vi "TEG P116x2w_Write_Auto.vi"(7 "MaxOutput":T1={"Ch1"=100.0, "Ch2"=100.0}, 8 "error in (no error)":errorcluster, 9 "RateSP":T1, 10 "NuevoSP":T1, 11 "Comunicaciones":T2={"Alicats"="ASRL6::INSTR", "Alic"=FALSE, "eValve"="ASRL6::INSTR", "eval"=FALSE, "Eurotherm"="ASRL6::INSTR", "euro"=FALSE, "Cell GAS"="ASRL6::INSTR", "cgas"=FALSE, "Cell H2S"="ASRL6::INSTR", "ch2s"=FALSE}) -> (0 "error out":errorcluster, 1 "RateSP(C/min) 2":T1, 2 "NuevoSP(C) 2":T1, 3 "MaxOutput 2":T1)   [LabVIEW 2017]
uses:
  2xP116.ctl
  REACTOR_COMUNICACIONES.ctl
  Eurotherm_2023_Module.ctl
  REACTOR_GLOBALES.vi
panel:
  out "Temp":T1
  in  "Cancel":bool
  in  "Write":bool
  out "Enable(T)":bool=TRUE
  out "VISA Promux":refnum<visa-resource-name>
  in  "Delay Time (s)":dbl=0.1
  # "Programando controladores P116"
  # "C"
  # "%"
  # "CALOR"
  # "C/min"
  # "C"
  # "%"
  # "FRIO"
  # "C/min"
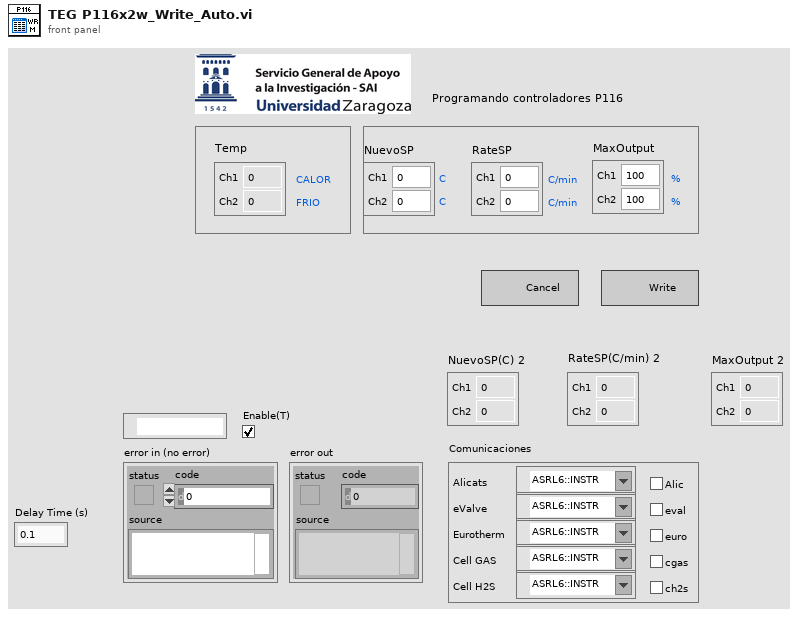
[diagram p1: front panel]
types:
  T1 = typedef "2xP116.ctl" = cluster{"Ch1":dbl, "Ch2":dbl}
  T2 = typedef "REACTOR_COMUNICACIONES.ctl" = cluster{"Alicats":refnum<visa-resource-name>, "Alic":bool, "eValve":refnum<visa-resource-name>, "eval":bool, "Eurotherm":refnum<visa-resource-name>, "euro":bool, "Cell GAS":refnum<visa-resource-name>, "cgas":bool, "Cell H2S":refnum<visa-resource-name>, "ch2s":bool}
  T3 = typedef "TEG P116x2w.ctl" = cluster{"TargetSP":T1, "WorkingSP":T1, "Temperatura":T1, "Error":bool, "Date":string, "Delay(s)":dbl, "RateSP":T1, "Potencia":T1, "Potencia max":T1}
  T4 = typedef "Eurotherm_2023_Module.ctl" = enum16{"Initialize", "Write setpoint", "Read data", "Write ramp rate", "Set constante proporcional", "Set constante integral", "Set constante diferencial", "Set ouput limit LOW", "Set ouput limit HIGH", "Shutdown"}
  T5 = enum16{"Add 1", "Add 2", "Add 3", "Add 10", "Add 11", "Add 12", "Add 13"}[]
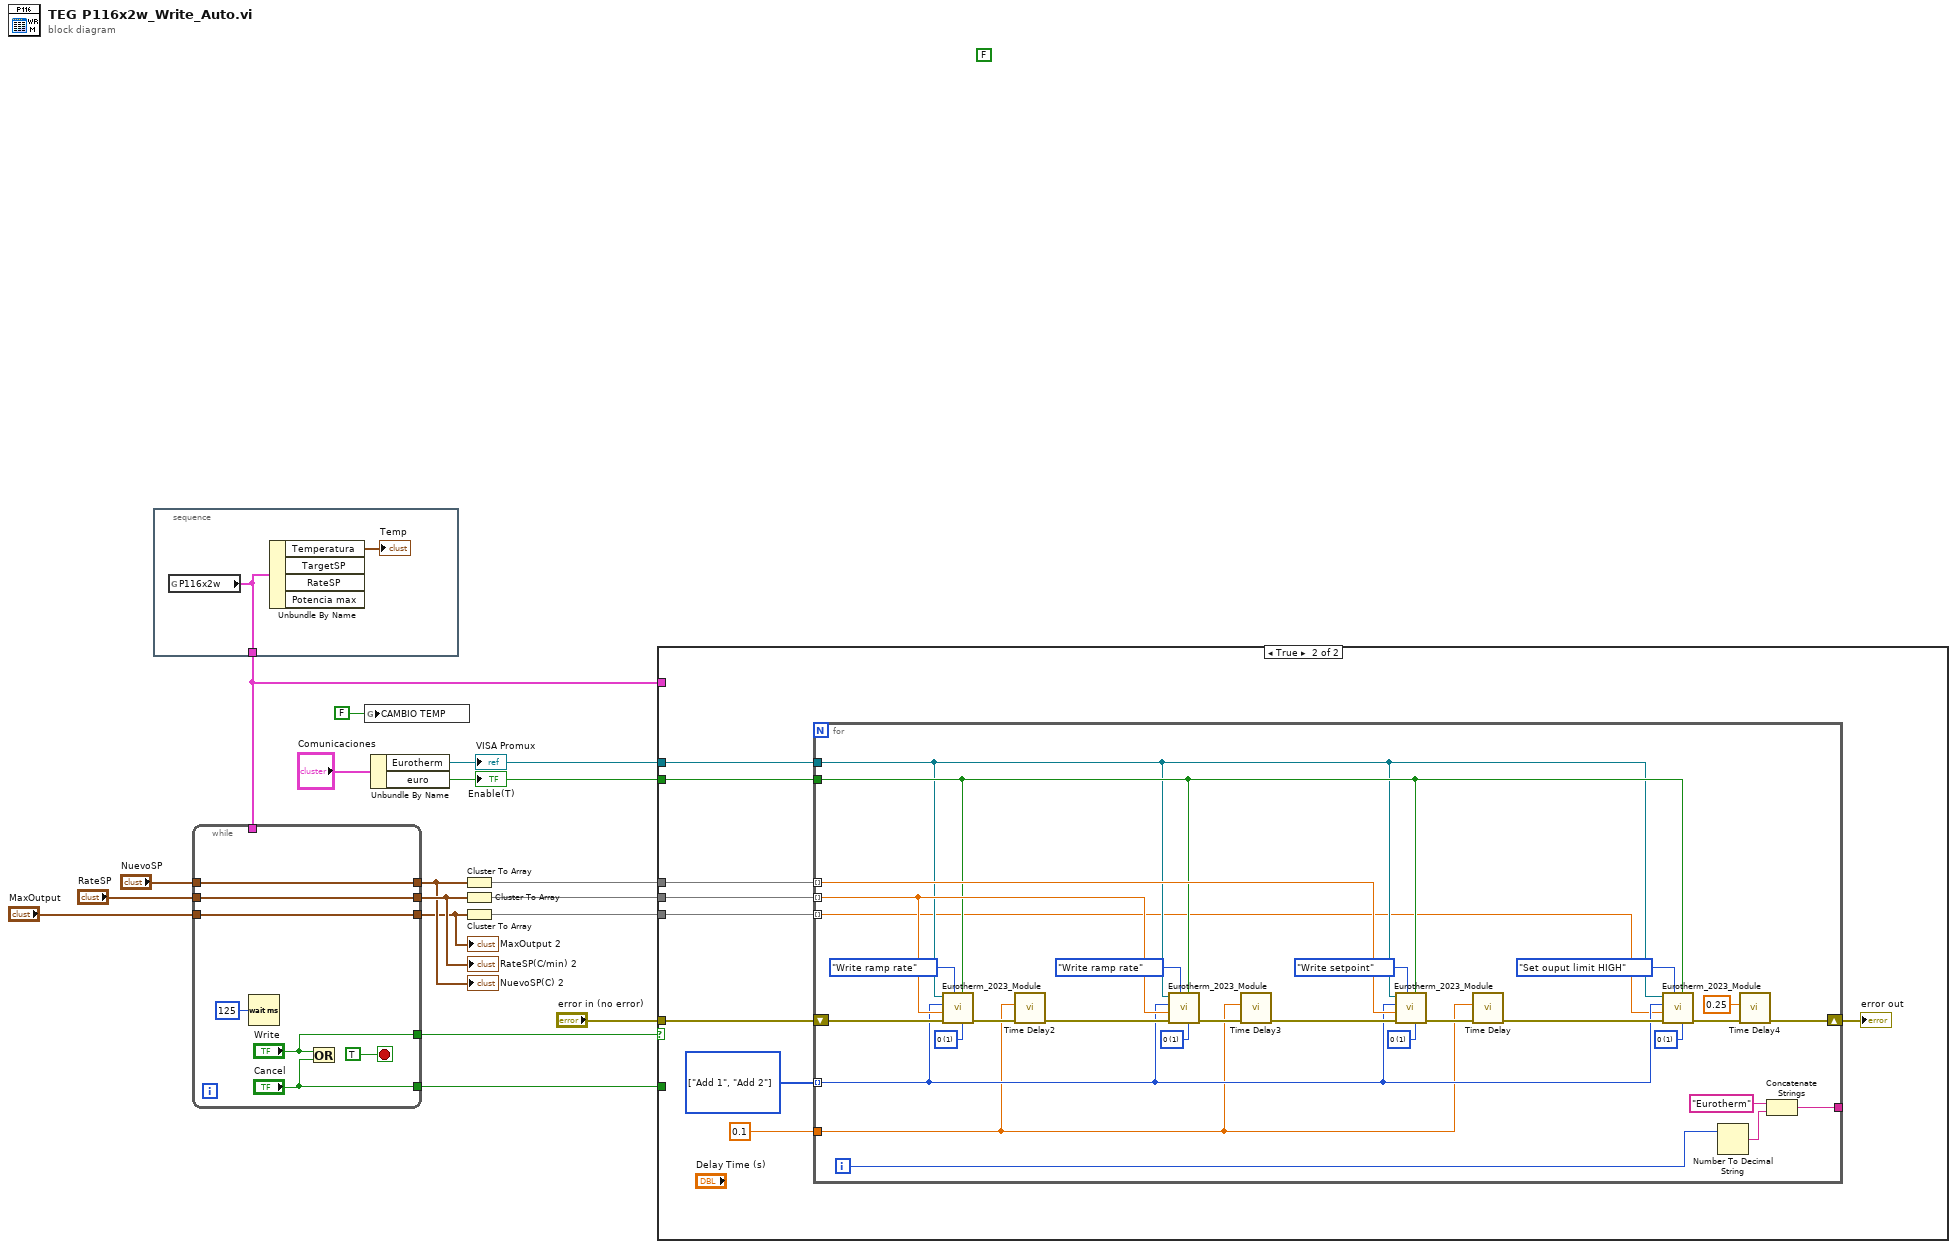
[diagram p0: block diagram]
diagram:
  (unwired) FALSE
  n1 = stacked-sequence {
    tunnel: [w18] -> w9
    frame #0 {
      n2 = global read "REACTOR_GLOBALES.vi" "P116x2w"() -> (w18:T3)
      n3 = Unbundle By Name(w18) -> ("Temperatura"=→"Temp":T1)  [unwired: 3 out]
    }
  }
  n4 = while {
    tunnel: ["Cancel"] -> w16
    tunnel: [w23] -> w5
    tunnel: [w22] -> w8
    tunnel: ["Write"] -> w12
    tunnel: w9 -> [_]
    tunnel: [w21] -> w4
    tunnel: "NuevoSP" -> [w23]
    tunnel: "RateSP" -> [w22]
    tunnel: "MaxOutput" -> [w21]
    stop <- TRUE stop-if-true
    n5 = Wait (ms)(milliseconds to wait=u32 125) -> ()  [unwired: 1 out]
    n6 = Or(x="Write", y="Cancel") -> ()  [unwired: 1 out]
  }
  "NuevoSP(C) 2" <- w5
  "RateSP(C/min) 2" <- w8
  "MaxOutput 2" <- w4
  n7 = global write "REACTOR_GLOBALES.vi" "CAMBIO TEMP"(FALSE ("ChangeT")) -> ()
  n8 = Unbundle By Name("Comunicaciones") -> ("Eurotherm"=w10:refnum<visa-resource-name>, "euro"=w17:bool)
  "Enable(T)" <- w17
  "VISA Promux" <- w10
  n9 = Cluster To Array(cluster=w5) -> (array=w14:dbl[])
  n10 = Cluster To Array(cluster=w8) -> (array=w13:dbl[])
  n11 = Cluster To Array(cluster=w4) -> (array=w6:dbl[])
  n12 = case shown="True" w12 {
    tunnel: w17 -> [_ w34]
    tunnel: w16 -> [_ _]
    tunnel: "error in (no error)" -> [_ w32]
    tunnel: w14 -> [_ w30]
    tunnel: w13 -> [_ w31]
    tunnel: w10 -> [_ w35]
    tunnel: w9 -> [_ _]
    tunnel: w6 -> [_ w28]
    frame False {
    }
    frame True {
      w29 = T5 [enum."Add 1", enum."Add 2"] items=["Add 1", "Add 2", "Add 3", "Add 10", "Add 11", "Add 12", "Add 13"]
      n13 = for {
        shift-right: [w42] -> w33
        shift-left: w32 -> [w59]
        tunnel: [w62] -> _
        tunnel: w30 -> [w58] mode=indexing
        tunnel: w31 -> [w47] mode=indexing
        tunnel: w35 -> [w40]
        tunnel: w34 -> [w41]
        tunnel: w29 -> [w39] mode=indexing
        tunnel: w28 -> [w36] mode=indexing
        tunnel: 0.1 ("Delay Time (s)") -> [w38]
        i -> [w56]
        w46 = u16 1 items=["0"=1, "1"=10, "2"=100] ("Decimales")
        w51 = u16 1 items=["0"=1, "1"=10, "2"=100] ("Decimales")
        w55 = u16 1 items=["0"=1, "1"=10, "2"=100] ("Decimales")
        w54 = u16 1 items=["0"=1, "1"=10, "2"=100] ("Decimales")
        n14 = call "Eurotherm_2023_Module.vi"("Decimales"=w55, "Eurotherm (T:Enable)"=w41, "Command"=Eurotherm_2023_Module."Write ramp rate", "error in (no error)"=w59, "Value"=w47, "Address"=w39, "VISA resource name"=w40) -> ("error out"=w53:errorcluster)  [unwired: 3 in, 1 out]
        n15 = call "Time Delay2"("error in (no error)"=w53, "Delay Time (s)"=w38) -> ("error out"=w49:errorcluster)  [unwired: 9 in]
        n16 = call "Eurotherm_2023_Module.vi"("Decimales"=w51, "Eurotherm (T:Enable)"=w41, "Command"=Eurotherm_2023_Module."Write ramp rate", "error in (no error)"=w49, "Value"=w47, "Address"=w39, "VISA resource name"=w40) -> ("error out"=w52:errorcluster)  [unwired: 3 in, 1 out]
        n17 = call "Time Delay3"("error in (no error)"=w52, "Delay Time (s)"=w38) -> ("error out"=w48:errorcluster)  [unwired: 9 in]
        n18 = call "Eurotherm_2023_Module.vi"("Decimales"=w54, "Eurotherm (T:Enable)"=w41, "Command"=Eurotherm_2023_Module."Write setpoint", "error in (no error)"=w48, "Value"=w58, "Address"=w39, "VISA resource name"=w40) -> ("error out"=w57:errorcluster)  [unwired: 3 in, 1 out]
        n19 = call "Time Delay"("error in (no error)"=w57, "Delay Time (s)"=w38) -> ("error out"=w43:errorcluster)  [unwired: 9 in]
        n20 = call "Eurotherm_2023_Module.vi"("Decimales"=w46, "Eurotherm (T:Enable)"=w41, "Command"=Eurotherm_2023_Module."Set ouput limit HIGH", "error in (no error)"=w43, "Value"=w36, "Address"=w39, "VISA resource name"=w40) -> ("error out"=w45:errorcluster)  [unwired: 3 in, 1 out]
        n21 = Number To Decimal String(number=w56) -> (decimal integer string=w63:string)  [unwired: 1 in]
        n22 = call "Time Delay4"("error in (no error)"=w45, "Delay Time (s)"=0.25) -> ("error out"=w42:errorcluster)  [unwired: 9 in]
        n23 = Concatenate Strings("Eurotherm" ("error source (\" \")"), w63) -> (w62:string)
      }
      "error out" <- w33
    }
  }
